vi "SHT21_Create.vi"(0 "reference in":refnum<class "SHT21.lvclass">, 2 "I2C Channel (0)":u8=1, 3 "I2C Slave Address (0)":u8, 5 "error in (no error)":errorcluster, 7 "T Offset":dbl, 9 "RH Offset":dbl) -> (14 "reference out":refnum<class "SHT21.lvclass">, 19 "error out":errorcluster)   [LabVIEW 2014, in "SHT21.lvclass"]
uses:
  SHT21.lvclass
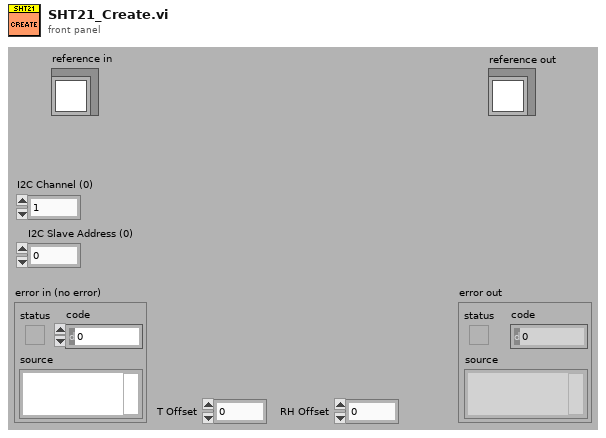
[diagram p1: front panel]
types:
  T1 = typedef "SHT21.lvclass/ObjectAttributes.ctl" = cluster{"I2C Slave Address":u8, "T Offset":dbl, "RH Offset":dbl, "I2C Channel":u8}
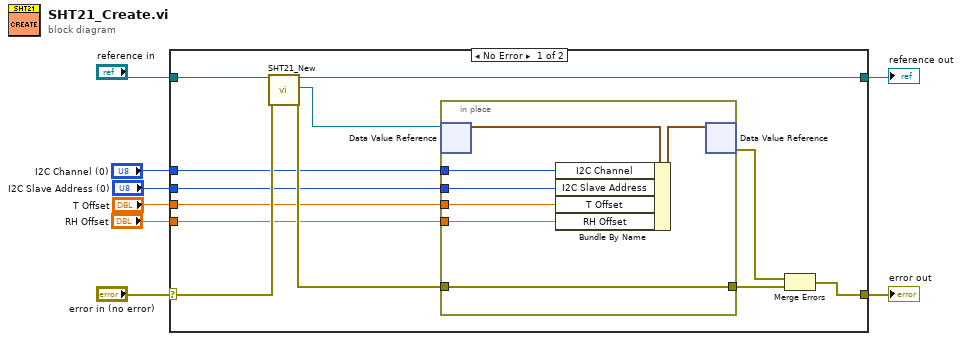
[diagram p0: block diagram]
diagram:
  n1 = case shown="No Error" "error in (no error)" {
    selector: "error in (no error)" -> [w19 w29]
    tunnel: [w16 w29] -> w7
    tunnel: "reference in" -> [w20 w28]
    tunnel: [w18 w28] -> w5
    tunnel: "I2C Slave Address (0)" -> [w12 _]
    tunnel: "T Offset" -> [w11 _]
    tunnel: "RH Offset" -> [w10 _]
    tunnel: "I2C Channel (0)" -> [w9 _]
    frame No Error {
      n2 = call "SHT21_New.vi"("reference in"=w20, "error in (no error)"=w19) -> ("reference out"=w18:refnum<class "SHT21.lvclass">, "DVRRefOut"=w15:refnum<data-value>, "error out"=w14:errorcluster)  [unwired: 14 in, 1 out]
      n3 = in-place {
        in-place-border: w14 -> [w25]
        in-place-border: [w25] -> w13
        in-place-border: w12 -> [w24]
        in-place-border: w11 -> [w23]
        in-place-border: w10 -> [w22]
        in-place-border: w9 -> [w21]
        n4 = in-place-dvr #1(w15) -> (w26:T1)  [unwired: 1 out]
        n5 = Bundle By Name(cluster=w26, "I2C Channel"=w21, "I2C Slave Address"=w24, "T Offset"=w23, "RH Offset"=w22) -> (w27:T1)
        n6 = in-place-dvr #1(w27) -> (w17:errorcluster)  [unwired: 1 out]
      }
      n7 = Merge Errors(w17, w13) -> (w16:errorcluster)
    }
    frame Error {
    }
  }
  "error out" <- w7
  "reference out" <- w5
